vi "Bool.vi"() -> ()   [LabVIEW 2018]
panel:
  out "x .implies. y?":bool
  out "x nand y":bool
  out "x xor y":bool
  out "x .or. y?":bool
  in  "불리언 2":bool
  in  "불리언":bool
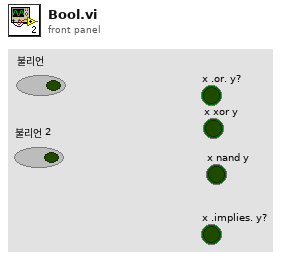
[diagram p1: front panel]
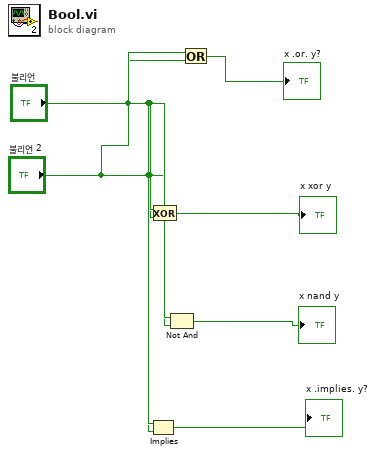
[diagram p0: block diagram]
diagram:
  n1 = Implies(1:"불리언 2", 2:"불리언") -> (0:→"x .implies. y?":bool)
  n2 = Exclusive Or(1:"불리언 2", 2:"불리언") -> (0:→"x xor y":bool)
  n3 = Not And(1:"불리언 2", 2:"불리언") -> (0:→"x nand y":bool)
  n4 = Or(x="불리언", y="불리언 2") -> (x .or. y?=→"x .or. y?":bool)
